vi "GetSpectrum.vi"() -> ()   [LabVIEW 2022 SP3]
panel:
  out "X":dbl[](array[numeric])
  in  "wavelength\ncoefficients":bool=TRUE
  out "XY Graph":cluster{"X":dbl[], dbl[]}[](graph)
  out "scan":i32
  out "Error":bool
  in  "keep trigger":bool
  in  "scans number":u8=1
  in  "N spectra (avrg)":u16=1
  in  "stop":bool
  in  "Exposure (*2.375 ms)":u16=2
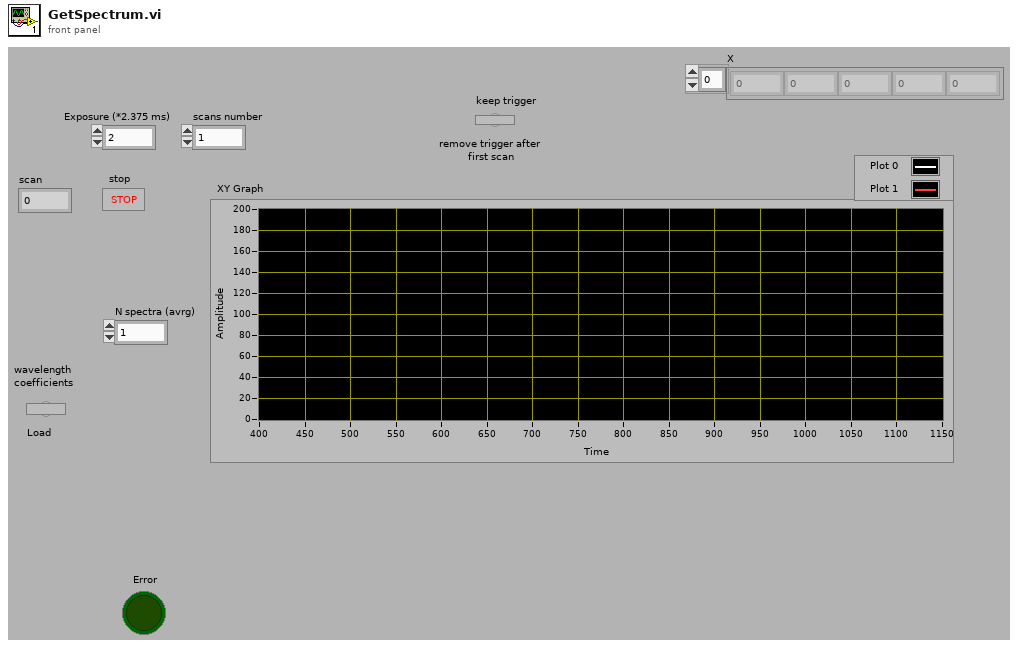
[diagram p1: front panel]
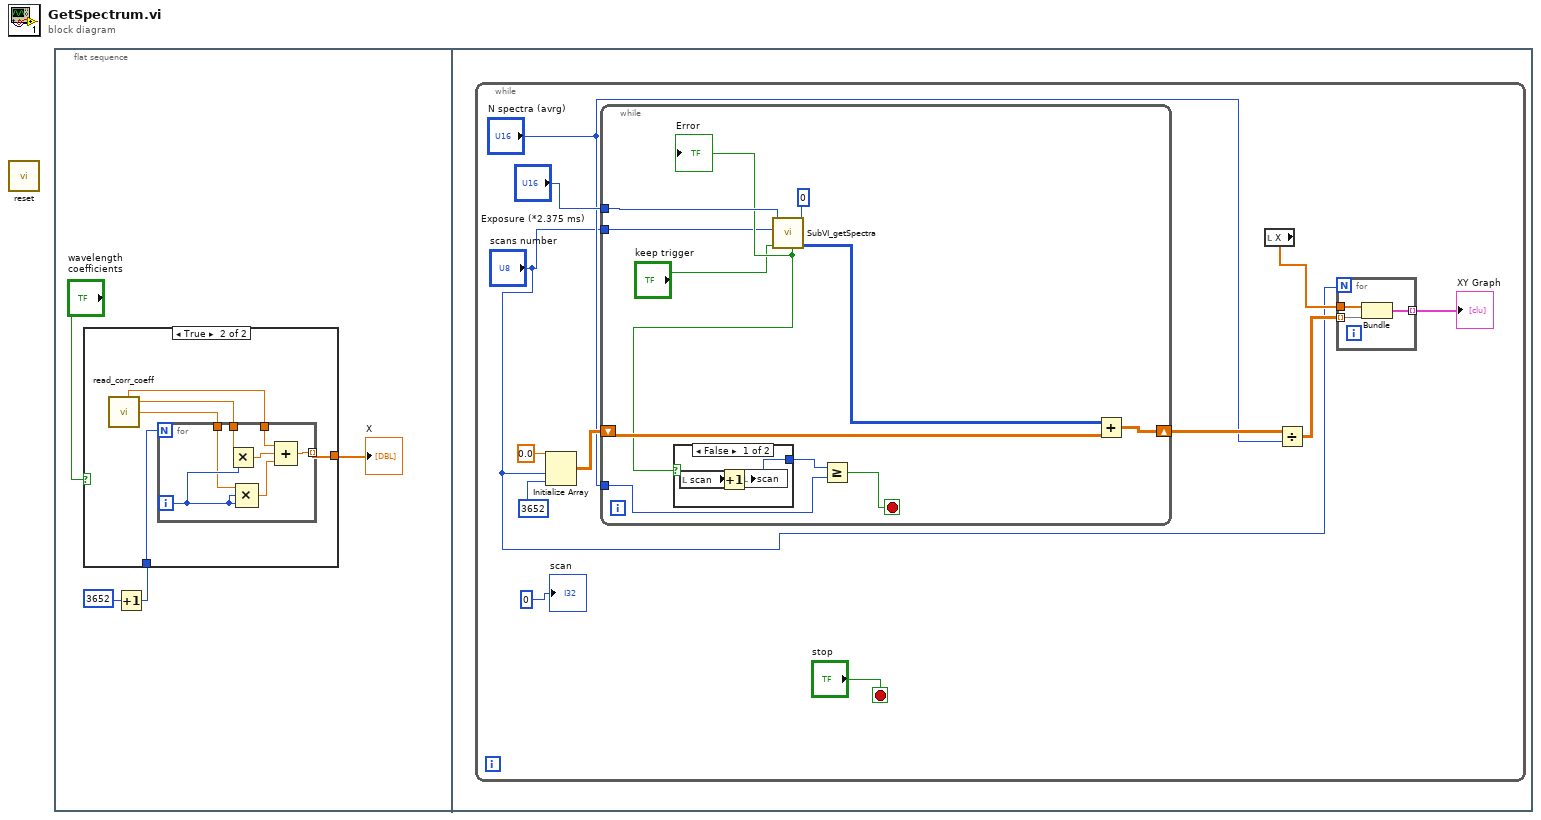
[diagram p0: block diagram]
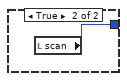
[diagram p3: hidden frame]
diagram:
  n1 = call "reset.vi"() -> ()  [unwired: 1 in]
  n2 = flat-sequence {
    frame #0 {
      n3 = Increment(x=u16 3652) -> (x+1=w3:u16)
      n4 = case shown="True" "wavelength\ncoefficients" {
        tunnel: w3 -> [w6 w11]
        tunnel: [w5 w12] -> w2
        frame False {
          n5 = for {
            N: w6 -> [_]
            tunnel: [w7] -> w5 mode=indexing
            i -> [w7]
          }
        }
        frame True {
          n6 = call "read_corr_coeff.vi"() -> ("A\n(Ax^2+Bx+C)"=w8:dbl, "B\n(Ax^2+Bx+C)"=w9:dbl, "C\n(Ax^2+Bx+C)"=w10:dbl)  [unwired: 1 in, 2 out]
          n7 = for {
            N: w11 -> [_]
            tunnel: w10 -> [w18]
            tunnel: w9 -> [w17]
            tunnel: w8 -> [w14]
            tunnel: [w16] -> w12 mode=indexing
            i -> [w15]
            n8 = Multiply(x=w17, y=w15) -> (x*y=w19:dbl)
            n9 = Compound Arithmetic op=MULTIPLY(w14, w15, w15) -> (w13:dbl)
            n10 = Compound Arithmetic op=ADD(w18, w19, w13) -> (w16:dbl)
          }
        }
      }
      "X" <- w2
    }
    frame #1 {
      n11 = while {
        stop <- "stop" stop-if-true
        n12 = Initialize Array(0.0 ("element"), "scans number", 3652 ("dimension size")) -> (w28:dbl[][])
        n13 = while {
          tunnel: "Exposure (*2.375 ms)" -> [w39]
          shift-right: [w44] -> w27
          shift-left: w28 -> [w45]
          tunnel: "N spectra (avrg)" -> [w41]
          tunnel: "scans number" -> [w36]
          stop <- w43 stop-if-true
          n14 = call "SubVI_getSpectra.vi"("test1"=u8 0, "keep trigger"="keep trigger", "scans number"=w36, "Exposure"=w39) -> ("all spectra"=w40:i16[][], "Error"=w37:bool)  [unwired: 6 in]
          "Error" <- w37
          n15 = case shown="False" w37 {
            tunnel: [w46 w48] -> w42
            frame False {
              n16 = local read "scan"() -> (w47:i32)
              n17 = Increment(x=w47) -> (x+1=w46:i32)
              n18 = local write "scan"(w46) -> ()
            }
            frame True {
              n19 = local read "scan"() -> (w48:i32)
            }
          }
          n20 = Greater Or Equal?(x=w42, y=w41) -> (x >= y?=w43:bool)
          n21 = Add(x=w40, y=w45) -> (x+y=w44:dbl[][])
        }
        n22 = local read "X"() -> (w24:dbl[])
        n23 = Divide(x=w27, y="N spectra (avrg)") -> (x/y=w25:dbl[][])
        n24 = for {
          N: "scans number" -> [_]
          tunnel: w24 -> [w34]
          tunnel: [w33] -> w26 mode=indexing
          tunnel: w25 -> [w32] mode=indexing
          n25 = Bundle("X"=w34, w32) -> (w33:cluster{"X":dbl[], dbl[]})  [unwired: 1 in]
        }
        "XY Graph" <- w26
        "scan" <- 0 ("current scan")
      }
    }
  }
